vi "6_3_1.vi"(9 "Map":map{string, refnum<vi>}(c390), 10 "Schlüssel":string[](array[string]), 11 "Deaktiviert":T1(array[ring])) -> ()   [LabVIEW 2020]
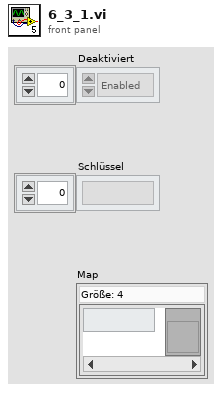
[diagram p1: front panel]
types:
  T1 = enum8{"Enabled", "Disabled", "Disabled and Grayed Out"}[]
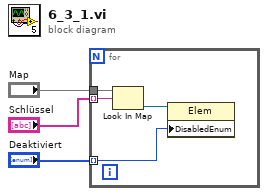
[diagram p0: block diagram]
diagram:
  n1 = for {
    tunnel: "Map" -> [w7]
    tunnel: "Schlüssel" -> [w6] mode=indexing
    tunnel: "Deaktiviert" -> [w4] mode=indexing
    n2 = Look In Map(map=w7, key=w6) -> (value=w5:refnum<vi>)  [unwired: 1 in, 1 out]
    n3 = property class="Elem"(reference=w5, "DisabledEnum"=w4) -> ()  [unwired: 1 in, 2 out]
  }
